vi "MyQH Error Handler - Event Handling Loop.vi"(8 "error in (no error)":T1 caption="Fehler (Eingang, kein Fehler)", 10 "Fehler ignorieren (Runtime)":i32[](array[numeric]), 11 "Nachrichten-Queue":refnum<queue>) -> (0 "Fehler (Eingang, Kopie)":T1, 3 "Nachrichten-Queue (Kopie)":refnum<queue>)   [LabVIEW 2014]
doc: "Reagiert auf Fehler in der Ereignisbehandlungsschleife, indem es die Fehler entweder ignoriert oder eine Fehlernachricht erzeugt."
uses:
  Message Queue/Message Cluster.ctl
  Message Queue/MyQH Message Queue.lvlib
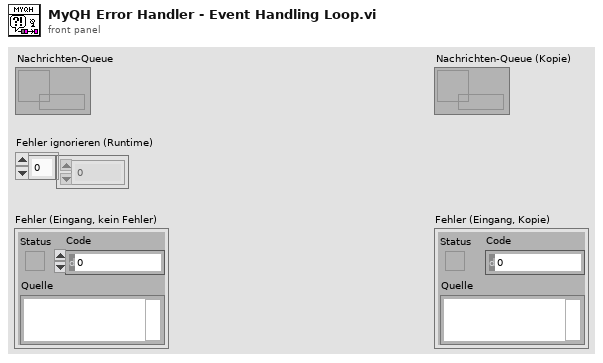
[diagram p1: front panel]
types:
  T1 = cluster{"Status":bool, "Code":i32, "Quelle":string}
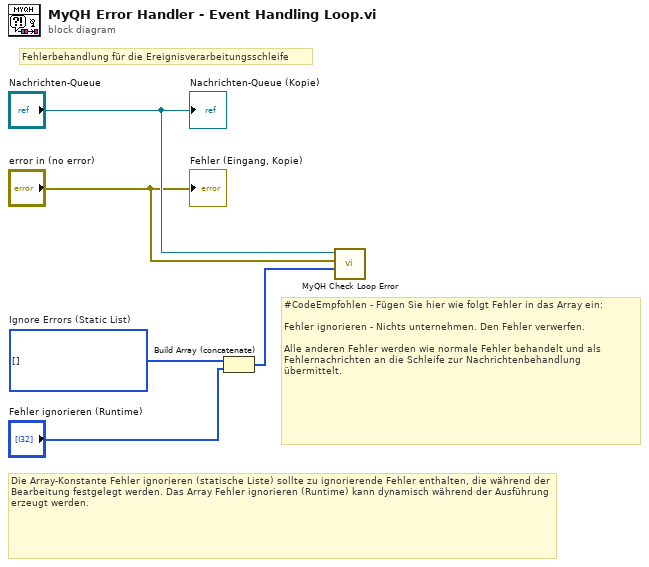
[diagram p0: block diagram]
diagram:
  w4 = i32[] []  # Ignore Errors (Static List)
  # "Die Array-Konstante Fehler ignorieren (statische Liste) sollte zu ignorierende Fehler enthalten, die während der Bearbeitung festgelegt werden. Das Array Fehler ignorieren (Runtime) kann dynamisch während der Ausführung erzeugt werden."
  # "#CodeEmpfohlen - Fügen Sie hier wie folgt Fehler in das Array ein:\n\nFehler ignorieren - Nichts unternehmen. Den Fehler verwerfen.\n\nAlle anderen Fehler werden wie normale Fehler behandelt und als Fehlernachrichten an die Schleife zur Nachrichtenbehandlung übermittelt."
  # "Fehlerbehandlung für die Ereignisverarbeitungsschleife"
  n1 = Build Array (concatenate)(w4, "Fehler ignorieren (Runtime)") -> (w3:i32[])
  n2 = call "MyQH Check Loop Error.vi"("Fehler ignorieren"=w3, "Zu verarbeitende Feher"="error in (no error)", "Nachrichten-Queue"="Nachrichten-Queue") -> ()  [unwired: 7 in, 2 out]
  "Nachrichten-Queue (Kopie)" <- "Nachrichten-Queue"
  "Fehler (Eingang, Kopie)" <- "error in (no error)"
